vi "load_data_file.vi"() -> ()   [LabVIEW 2011]
panel:
  in  "Create Pulse":bool
  in  "Backup Directory":path=path "Z:/usb650_d_tmp_data"
  in  "Data Comments":string
  in  "File Type":i32(listbox)
  in  "Data File":path
  in  "Shot Date":timestamp format="%<%x>T"
  in  "stop":bool
  in  "Run #":i32
  in  "Generate New Shot Number":bool
  in  "MDSPlus Host":string="shanghai.ph.utexas.edu"
  in  "Tree":string="machine"
  in  "Load Data":bool
  in  "New Shot Number":i32
  # "Please use stop button to terminate program."
  # "MDSPlus Settings"
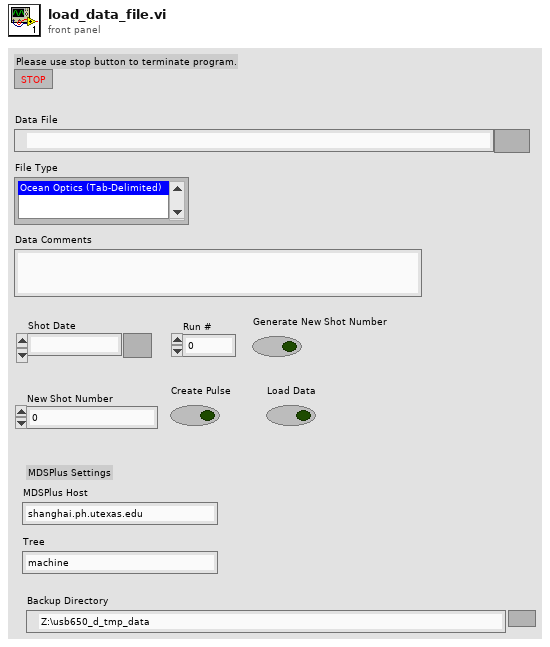
[diagram p1: front panel]
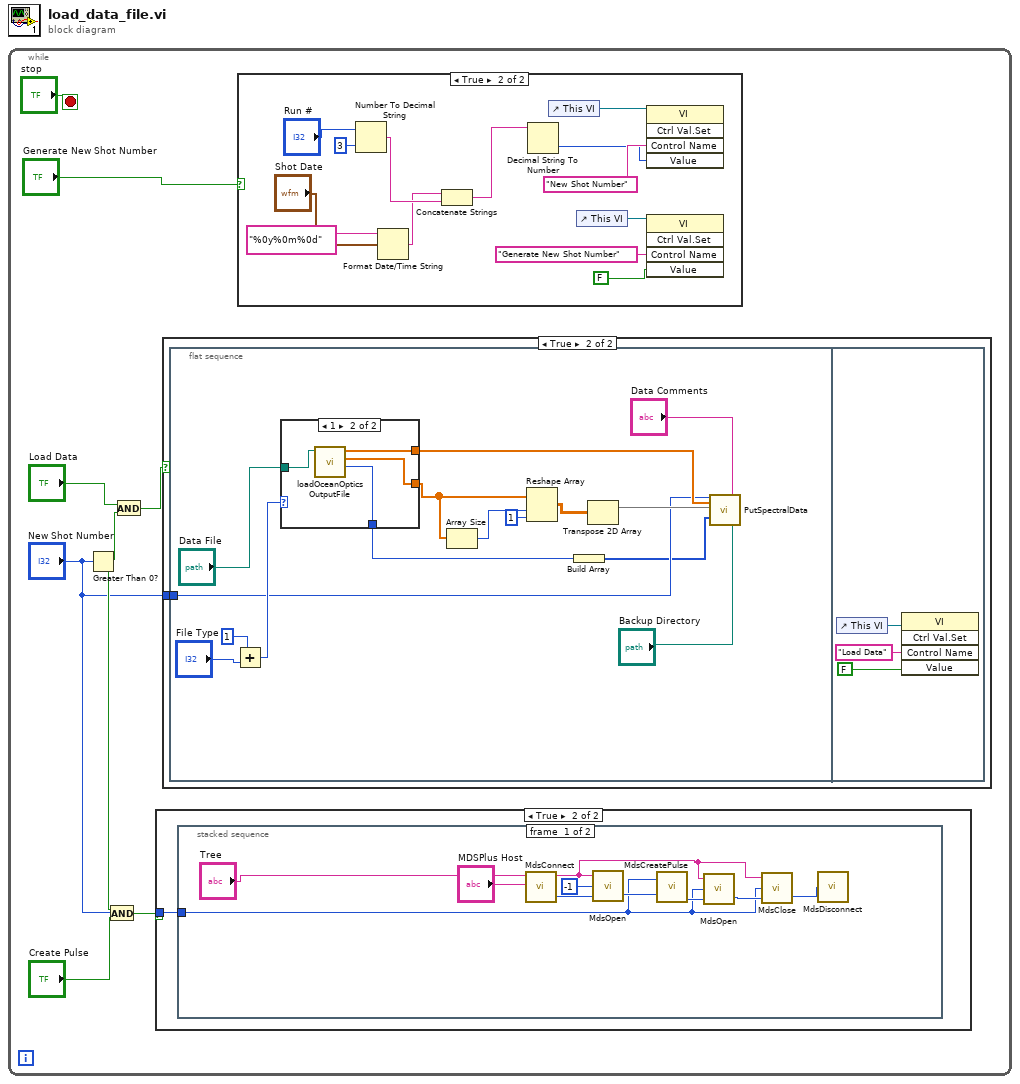
[diagram p0: block diagram]
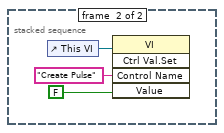
[diagram p3: hidden frame]
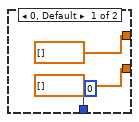
[diagram p5: hidden frame]
diagram:
  n1 = while {
    stop <- "stop" stop-if-true
    n2 = Greater Than 0?(x="New Shot Number") -> (x > 0?=w3:bool)
    n3 = And(x=w3, y="Create Pulse") -> (x .and. y?=w4:bool)
    n4 = And(x="Load Data", y=w3) -> (x .and. y?=w5:bool)
    n5 = case shown="True" w4 {
      tunnel: "New Shot Number" -> [_ w9]
      frame False {
      }
      frame True {
        n6 = stacked-sequence {
          tunnel: w9 -> [w10 _]
          frame #0 {
            n7 = call "MdsConnect.vi"("Host"="MDSPlus Host") -> ("FlowControlOut"=w14:i32)  [unwired: 1 in, 1 out]
            n8 = call "MdsOpen.vi"("FlowControlIn"=w14, "Shot"=-1, "Tree"="Tree") -> ("FlowControlOut"=w15:i32)  [unwired: 1 out]
            n9 = call "MdsCreatePulse.vi"("FlowControlIn"=w15, "Shot Number"=w10) -> ("FlowControlOut"=w16:i32)  [unwired: 1 in]
            n10 = call "MdsOpen.vi"("FlowControlIn"=w16, "Shot"=w10, "Tree"="Tree") -> ("FlowControlOut"=w11:i32)  [unwired: 1 out]
            n11 = call "MdsClose.vi"("FlowControlIn"=w11, "Shot"=w10, "Tree"="Tree") -> ("FlowControlOut"=w18:i32)  [unwired: 1 out]
            n12 = call "MdsDisconnect.vi"("FlowControlIn"=w18) -> ()  [unwired: 1 out]
          }
          frame #1 {
            n13 = control-ref of="This VI"() -> (w19:refnum<vi>)
            n14 = invoke class="VI" method="Ctrl Val.Set"(reference=w19, "Control Name"="Create Pulse", "Value"=FALSE) -> ()  [unwired: 2 in, 5 out]
          }
        }
      }
    }
    n15 = case shown="True" w5 {
      tunnel: "New Shot Number" -> [_ w22]
      frame False {
      }
      frame True {
        n16 = flat-sequence {
          tunnel: w22 -> [w27]
          frame #0 {
            n17 = Add(x=1, y="File Type") -> (x+y=w35:i32)
            n18 = case shown="1" w35 {
              tunnel: "Data File" -> [_ w44]
              tunnel: [dbl[] [] ("Counts") w43] -> w33
              tunnel: [dbl[] [] ("wavelengths") w42] -> w28
              tunnel: [0 ("IntegrationTime") w41] -> w26
              frame 0, Default {
              }
              frame 1 {
                n19 = call "loadOceanOpticsOutputFile.vi"("File"=w44) -> ("IntegrationTime"=w41:i32, "Counts"=w43:dbl[], "wavelengths"=w42:dbl[])  [unwired: 8 in]
              }
            }
            n20 = Array Size(array=w33) -> (size(s)=w32:i32)
            n21 = Reshape Array(w33, w32, 1 ("dimension size")) -> (w30:dbl[][])
            n22 = Build Array(w26) -> (w25:i32[])
            n23 = Transpose 2D Array(2D array=w30) -> (transposed array=w29:dbl[][])
            n24 = call "PutSpectralData.vi"("shot"=w27, "wavelengths"=w28, "Counts"=w29, "Integration Times"=w25, "Comments"="Data Comments", "backup_directory"="Backup Directory") -> ()  [unwired: 14 in]
          }
          frame #1 {
            n25 = control-ref of="This VI"() -> (w45:refnum<vi>)
            n26 = invoke class="VI" method="Ctrl Val.Set"(reference=w45, "Control Name"="Load Data", "Value"=FALSE) -> ()  [unwired: 2 in, 5 out]
          }
        }
      }
    }
    n27 = case shown="True" "Generate New Shot Number" {
      frame False {
      }
      frame True {
        n28 = Number To Decimal String(number="Run #", width (-)=i16 3) -> (decimal integer string=w57:string)
        n29 = Format Date/Time String(time format string (%c)="%0y%0m%0d", seconds (now)="Shot Date") -> (date/time string=w53:string)  [unwired: 1 in]
        n30 = Concatenate Strings(w53, w57) -> (w52:string)
        n31 = Decimal String To Number(string=w52) -> (number=w54:i32)  [unwired: 2 in, 1 out]
        n32 = control-ref of="This VI"() -> (w56:refnum<vi>)
        n33 = control-ref of="This VI"() -> (w51:refnum<vi>)
        n34 = invoke class="VI" method="Ctrl Val.Set"(reference=w56, "Control Name"="New Shot Number", "Value"=w54) -> ()  [unwired: 2 in, 5 out]
        n35 = invoke class="VI" method="Ctrl Val.Set"(reference=w51, "Control Name"="Generate New Shot Number", "Value"=FALSE) -> ()  [unwired: 2 in, 5 out]
      }
    }
  }
